vi "4155C Config V Stress.vi"(0 "VISA session":refnum<visa-resource-name>, 1 "ID compliance":dbl min=0.0 max=100000000000.0 format="%.15e", 2 "VD":dbl min=0.0 max=100000000000.0 format="%.15e", 3 "VG":dbl min=0.0 max=100000000000.0 format="%.15e", 4 "IG compliance":dbl min=0.0 max=100000000000.0 format="%.15e", 5 "error in (no error)":errorcluster, 7 "Display on/off":bool) -> (6 "dup VISA resource name":refnum<visa-resource-name>, 8 "error out":errorcluster)   [LabVIEW 2016]
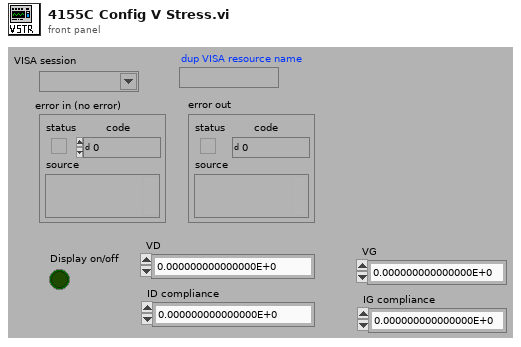
[diagram p1: front panel]
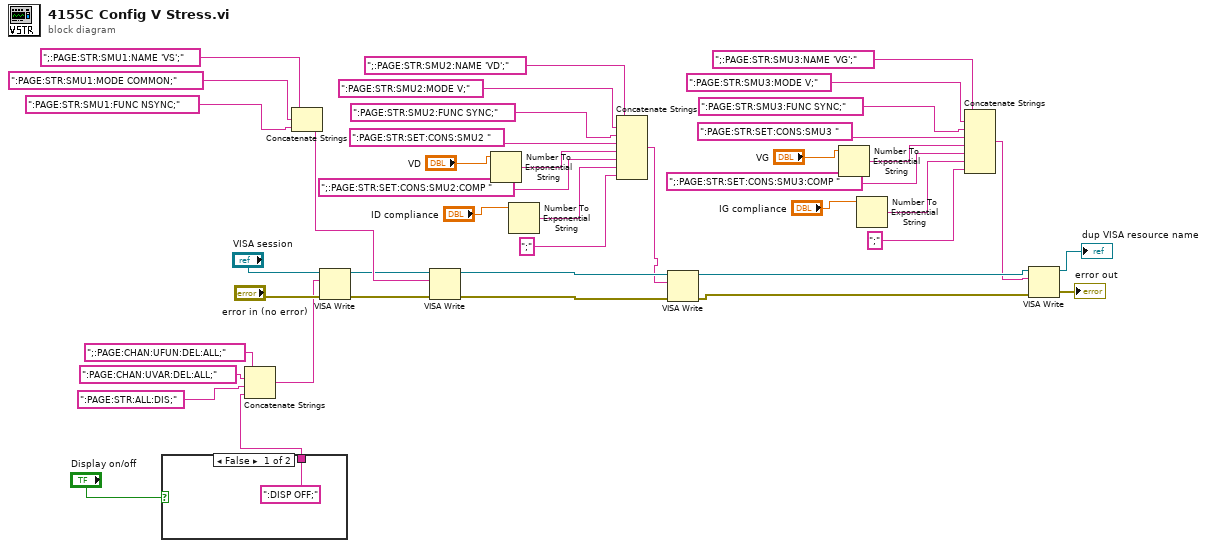
[diagram p0: block diagram]
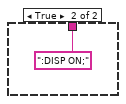
[diagram p2: hidden frame]
diagram:
  n1 = case shown="False" "Display on/off" {
    tunnel: [":DISP OFF;" ("write buffer (\"\")") ":DISP ON;" ("write buffer (\"\")")] -> w36
    frame False {
    }
    frame True {
    }
  }
  n2 = Concatenate Strings(";:PAGE:CHAN:UFUN:DEL:ALL;", ":PAGE:CHAN:UVAR:DEL:ALL;", ":PAGE:STR:ALL:DIS;", w36) -> (w37:string)
  n3 = Concatenate Strings(";:PAGE:STR:SMU1:NAME 'VS';", ":PAGE:STR:SMU1:MODE COMMON;", ":PAGE:STR:SMU1:FUNC NSYNC;") -> (w9:string)
  n4 = VISA Write(VISA resource name="VISA session", write buffer=w37, error in (no error)="error in (no error)") -> (VISA resource name out=w8:refnum<visa-resource-name>, error out=w7:errorcluster)  [unwired: 1 out]
  n5 = VISA Write(VISA resource name=w8, write buffer=w9, error in (no error)=w7) -> (VISA resource name out=w42:refnum<visa-resource-name>, error out=w41:errorcluster)  [unwired: 1 out]
  n6 = Number To Exponential String(number="VD") -> (E-format string=w24:string)  [unwired: 3 in]
  n7 = Number To Exponential String(number="ID compliance") -> (E-format string=w22:string)  [unwired: 3 in]
  n8 = Concatenate Strings(";:PAGE:STR:SMU2:NAME 'VD';", ":PAGE:STR:SMU2:MODE V;", ":PAGE:STR:SMU2:FUNC SYNC;", ":PAGE:STR:SET:CONS:SMU2 ", w24, ";:PAGE:STR:SET:CONS:SMU2:COMP ", w22, ";" ("Substring")) -> (w6:string)
  n9 = VISA Write(VISA resource name=w42, write buffer=w6, error in (no error)=w41) -> (VISA resource name out=w4:refnum<visa-resource-name>, error out=w5:errorcluster)  [unwired: 1 out]
  n10 = Number To Exponential String(number="VG") -> (E-format string=w14:string)  [unwired: 3 in]
  n11 = Number To Exponential String(number="IG compliance") -> (E-format string=w12:string)  [unwired: 3 in]
  n12 = Concatenate Strings(";:PAGE:STR:SMU3:NAME 'VG';", ":PAGE:STR:SMU3:MODE V;", ":PAGE:STR:SMU3:FUNC SYNC;", ":PAGE:STR:SET:CONS:SMU3 ", w14, ";:PAGE:STR:SET:CONS:SMU3:COMP ", w12, ";" ("Substring")) -> (w3:string)
  n13 = VISA Write(VISA resource name=w4, write buffer=w3, error in (no error)=w5) -> (VISA resource name out=→"dup VISA resource name":refnum<visa-resource-name>, error out=→"error out":errorcluster)  [unwired: 1 out]
